vi "Test_Common To All Boards.vi"(1 "board image":T2) -> (0 "pass?":T1)   [LabVIEW 2023]
doc: "Image check for blocks that are common to all types of boards."
uses:
  Common/Board Image.ctl
  Common/Pass Fail Boolean.ctl
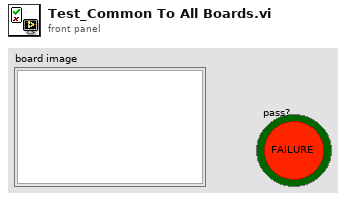
[diagram p1: front panel]
types:
  T1 = typedef "Pass Fail Boolean.ctl" = bool
  T2 = typedef "Board Image.ctl" = picture
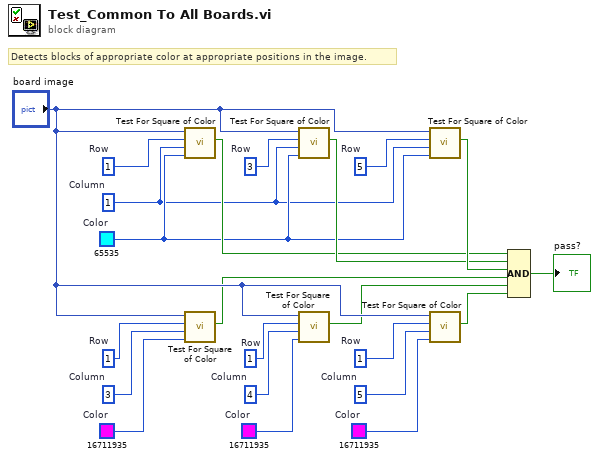
[diagram p0: block diagram]
diagram:
  w13 = i16 5  # Column
  w14 = i16 1  # Row
  w12 = u32 16711935  # Color
  w10 = i16 4  # Column
  w9 = i16 1  # Row
  w11 = u32 16711935  # Color
  w7 = i16 3  # Column
  w8 = i16 1  # Row
  w6 = u32 16711935  # Color
  w3 = i16 5  # Row
  w2 = i16 3  # Row
  w4 = i16 1  # Column
  w1 = i16 1  # Row
  w5 = u32 65535  # Color
  # "Detects blocks of appropriate color at appropriate positions in the image."
  n1 = call "Test For Square of Color.vi"("color"=w5, "column"=w4, "row"=w1, "board image"="board image") -> ("pass?"=w15:T1)  [unwired: 7 in]
  n2 = call "Test For Square of Color.vi"("color"=w6, "column"=w7, "row"=w8, "board image"="board image") -> ("pass?"=w18:T1)  [unwired: 7 in]
  n3 = call "Test For Square of Color.vi"("color"=w5, "column"=w4, "row"=w2, "board image"="board image") -> ("pass?"=w16:T1)  [unwired: 7 in]
  n4 = call "Test For Square of Color.vi"("color"=w11, "column"=w10, "row"=w9, "board image"="board image") -> ("pass?"=w19:T1)  [unwired: 7 in]
  n5 = call "Test For Square of Color.vi"("color"=w5, "column"=w4, "row"=w3, "board image"="board image") -> ("pass?"=w17:T1)  [unwired: 7 in]
  n6 = call "Test For Square of Color.vi"("color"=w12, "column"=w13, "row"=w14, "board image"="board image") -> ("pass?"=w20:T1)  [unwired: 7 in]
  n7 = Compound Arithmetic op=AND(w15, w16, w17, w18, w19, w20) -> (→"pass?":T1)
